vi "Get Message Name.vi"(8 "error in":errorcluster, 11 "message in":T1 format="%.0x") -> (0 "error out":errorcluster, 2 "message name":string, 3 "message out":T1 format="%.0x", 4 "found?":bool)   [LabVIEW 2020, in "Ballard MIL-STD-1553 Scripting.lvlib"]
doc: "Reads the <b>description</b> field of the input <b>Ballard MIL-STD 1553 custom device</b>."
uses:
  Ballard MIL-STD-1553 Scripting.lvlib
  <vilib>/NI VeriStand/Custom Device API/Custom Device Item Ref.ctl
  Constants.vi
  <vilib>/NI VeriStand/Custom Device API/Get Item Property (String).vi
  <vilib>/NI VeriStand/Custom Device API/Custom Device API.lvlib
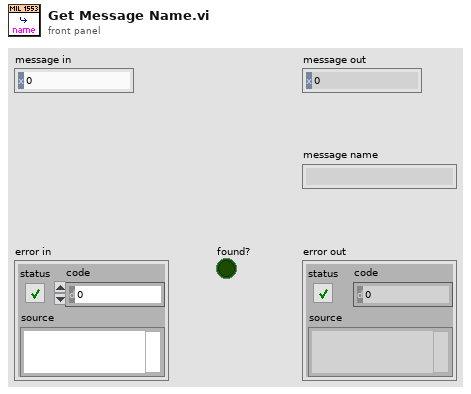
[diagram p1: front panel]
types:
  T1 = typedef "Custom Device API.lvlib/Custom Device Item Ref.ctl" = u64
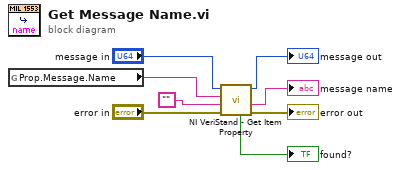
[diagram p0: block diagram]
diagram:
  n1 = global read "Constants.vi" "Prop.Message.Name"() -> (w2:string)
  n2 = call-poly <vilib>:"NI VeriStand - Get Item Property.vi"("error in (no error)"="error in", "Default Value"="", "Property Name"=w2, "Item Ref in"="message in") -> ("error out"=→"error out":errorcluster, "Value"=→"message name":string, "Item Ref out"=→"message out":T1, "Found?"=→"found?":bool)  [unwired: 4 in]
